vi "Read Stamp Slots.vi"(8 "error in (no error)":errorcluster, 11 "WorkTable Class in":refnum<class "WorkTable Class.lvclass">) -> (0 "error out":errorcluster, 2 "Stamp Slots":T1(array[cluster]), 3 "WorkTable Class out":refnum<class "WorkTable Class.lvclass">)   [LabVIEW 2011, in "WorkTable Class.lvclass"]
uses:
  WorkTable Class.lvclass
  WorkTable Class.lvclass/WorkTable Class.ctl
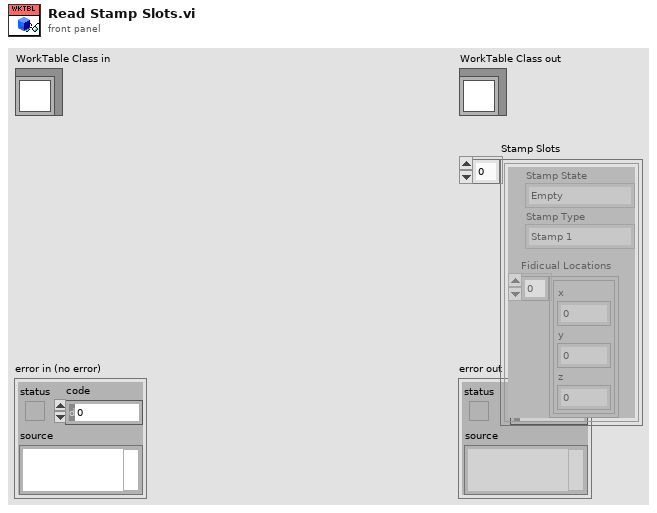
[diagram p1: front panel]
types:
  T1 = cluster{"Stamp State":enum16{"Empty", "Populated", "Used"}, "Stamp Type":enum16{"Stamp 1", "Stamp 2", "Stamp 3", "Stamp 4"}, "Fidicual Locations":cluster{"x":dbl, "y":dbl, "z":dbl}[]}[]
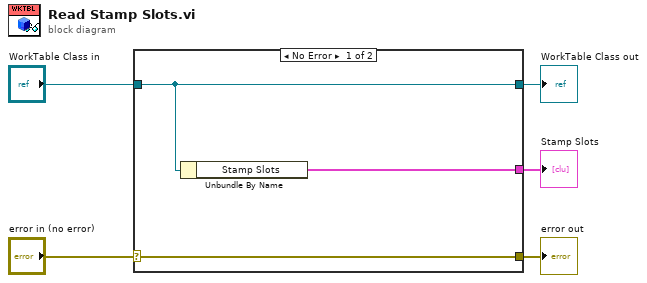
[diagram p0: block diagram]
diagram:
  n1 = case shown="No Error" "error in (no error)" {
    selector: "error in (no error)" -> [w8 w9]
    tunnel: [w8 w9] -> w4
    tunnel: [w7 w10] -> w2
    tunnel: "WorkTable Class in" -> [w7 w10]
    tunnel: [w6 _] -> w1
    frame No Error {
      n2 = Unbundle By Name(w7) -> ("Stamp Slots"=w6:T1)
    }
    frame Error {
    }
  }
  "error out" <- w4
  "WorkTable Class out" <- w2
  "Stamp Slots" <- w1
